vi "Limiter-WL Input.vi"(1 "Current Grating Density":enum16{"150", "300", "600", "1200", "1800"}(ring)=enum."1200" caption="Grating Density", 2 "Central WL Input":dbl=619.92122 format="%.4f", 3 "X-Axis":i32(ring)=1 items=["Point #", "nm", "eV", "meV", "cm-1"]) -> (0 "Central WL output":dbl=619.92122 format="%.4f")   [LabVIEW 2020]
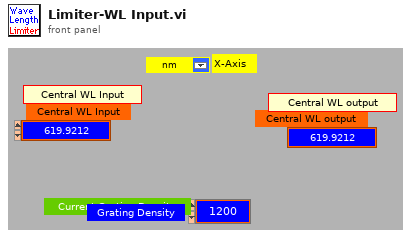
[diagram p1: front panel]
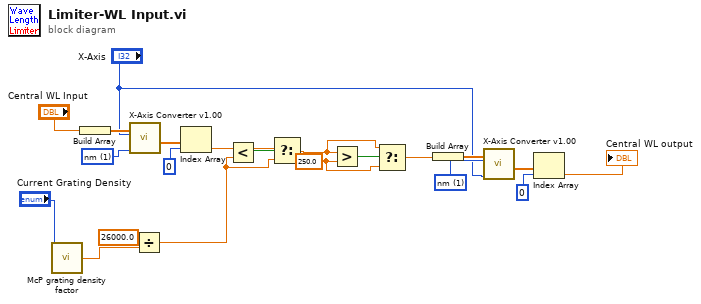
[diagram p0: block diagram]
diagram:
  w4 = 250.0 ("y")
  w8 = 1 items=["Point #", "nm", "eV", "meV", "cm-1"] ("X-Axis Unit")
  w19 = 1 items=["Point #", "nm", "eV", "meV", "cm-1"] ("X-Axis Unit")
  n1 = call "McP grating density factor.vi"("Grating Density"="Current Grating Density") -> ("GratingFactor"=w2:dbl)
  n2 = Build Array("Central WL Input") -> (w20:dbl[])
  n3 = call "X-Axis Converter v1.00.vi"("X-Axis Unit"=w19, "Old X-Axis Unit"="X-Axis", "X-Axis input"=w20) -> ("X-Axis Output"=w17:dbl[])  [unwired: 2 in, 3 out]
  n4 = Divide(x=26000.0, y=w2) -> (x/y=w13:dbl)
  n5 = Index Array(array=w17, index=0) -> (element=w14:dbl)
  n6 = Less?(x=w14, y=w13) -> (x < y?=w15:bool)
  n7 = Select(t=w14, s=w15, f=w13) -> (s? t:f=w5:dbl)
  n8 = Greater?(x=w5, y=w4) -> (0:w6:bool)
  n9 = Select(t=w5, s=w6, f=w4) -> (s? t:f=w3:dbl)
  n10 = Build Array(w3) -> (w12:dbl[])
  n11 = call "X-Axis Converter v1.00.vi"("X-Axis Unit"="X-Axis", "Old X-Axis Unit"=w8, "X-Axis input"=w12) -> ("X-Axis Output"=w11:dbl[])  [unwired: 2 in, 3 out]
  n12 = Index Array(array=w11, index=0) -> (element=→"Central WL output":dbl)
